vi "Read Payload.vi"(11 "ActionStack in":refnum<class "Action.lvclass">) -> (2 "Payload":variant, 3 "ActionStack out":refnum<class "Action.lvclass">)   [LabVIEW 2024, in "ActionStack.lvlib" / "Action.lvclass"]
uses:
  Action.lvclass
  Action.lvclass/Action.ctl
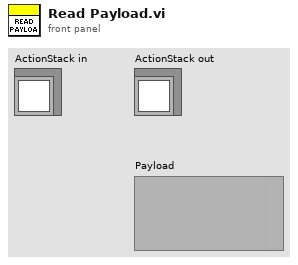
[diagram p1: front panel]
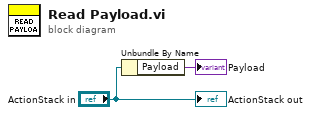
[diagram p0: block diagram]
diagram:
  n1 = Unbundle By Name("ActionStack in") -> ("Payload"=→"Payload":variant)
  "ActionStack out" <- "ActionStack in"
